vi "deflection reverse control.vi"() -> ()   [LabVIEW 2017]
uses:
  <vilib>/rvi/Emulation/niFpgaGetClockAttributes.vi
  <vilib>/rvi/Emulation/niFpgaSctlEmulationGetInTimedLoop.vi
  <vilib>/rvi/Emulation/niFpgaEmulationReportErrorSimple.vi
  <vilib>/rvi/eio/common/nirviEmuTemplateMethod_errors.vi
  <vilib>/rvi/Emulation/niFpgaCriticalErrorInLSC.vi
  <vilib>/eio/EIONode/EIONode.xnode
  <vilib>/rvi/FXPMathLib/FxpSub/XNode/nifxpmath_Sub.xnode
  <vilib>/rvi/FXPMathLib/FxpMul/XNode/nifxpmath_Multiplier.xnode
  <vilib>/rvi/FXPMathLib/FxpAdd/XNode/nifxpmath_Add.xnode
  <vilib>/rvi/FXPMathLib/sim/FxpSim.dll
panel:
  out "z sensor":fxp<+/-,20,5>
  in  "Lower Limit":fxp<+/-,64,29>=-8.0
  in  "Upper Limit":fxp<+/-,64,29>=8.0
  in  "P":fxp<+/-,20,5>=0.04998779296875
  in  "I":fxp<+/-,20,5>=0.029998779296875
  in  "SetPoint":fxp<+/-,20,5>
  in  "stop":bool
  out "deflection sensor":fxp<+/-,20,5>=0.018218994140625
  out "Output":fxp<+/-,64,29>=-1.1850092191016302
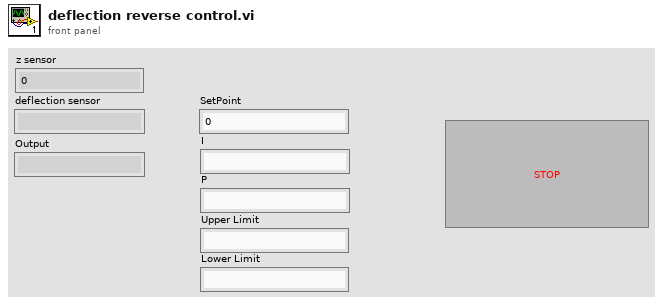
[diagram p1: front panel]
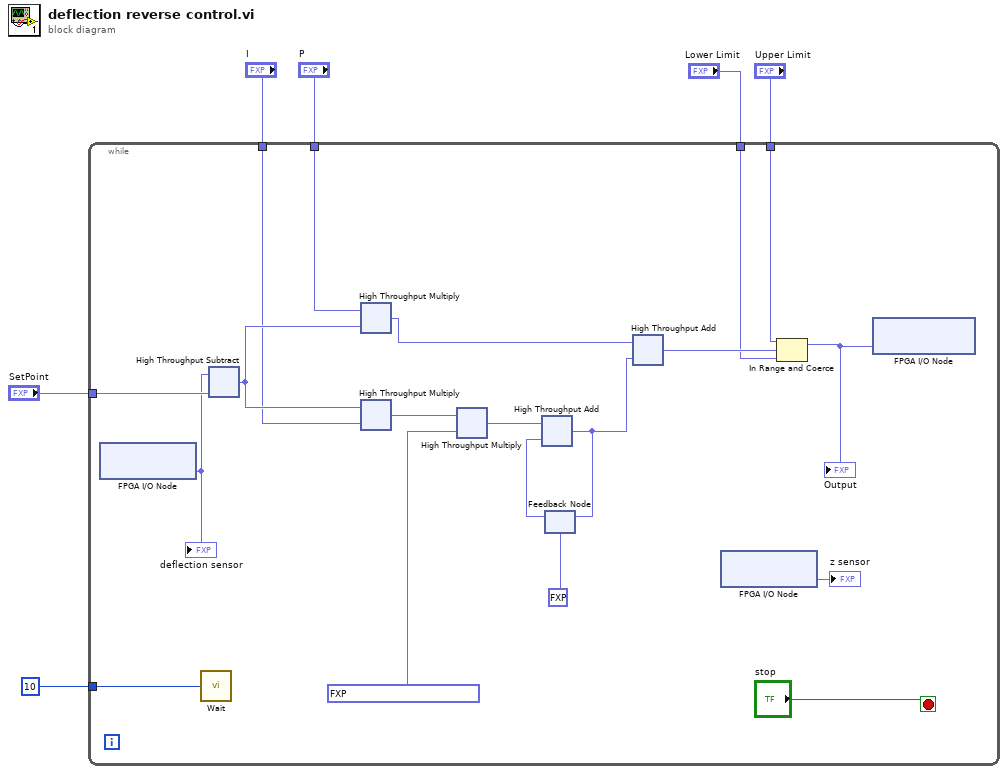
[diagram p0: block diagram]
diagram:
  n1 = while {
    tunnel: "SetPoint" -> [w9]
    tunnel: "P" -> [w24]
    tunnel: "I" -> [w22]
    tunnel: u32 10 ("Count(uSec)") -> [w20]
    tunnel: "Upper Limit" -> [w12]
    tunnel: "Lower Limit" -> [w11]
    stop <- "stop" stop-if-true
    n2 = xnode "FPGA I/O Node"() -> ("Mod1/AI3"=w8:fxp<+/-,20,5>)  [unwired: 1 in, 1 out]
    "deflection sensor" <- w8
    n3 = call "Wait"("Count(uSec)"=w20) -> ()  [unwired: 1 out]
    n4 = xnode ("High Throughput Subtract")("x"=w8, "y"=w9) -> ("x-y"=w23:fxp<+/-,21,6>)
    n5 = xnode ("High Throughput Multiply")("x"=w24, "y"=w23) -> ("x*y"=w15:fxp<+/-,41,11>)
    n6 = xnode ("High Throughput Multiply")("x"=w23, "y"=w22) -> ("x*y"=w21:fxp<+/-,41,11>)
    n7 = xnode ("High Throughput Multiply")("x"=w21, "y"=fxp<+/-,32,5> 9.998679161071777e-06) -> ("x*y"=w18:fxp<+/-,64,16>)
    n8 = feedback #1(fxp<+,1,1> 0.0) -> (w16:fxp<+/-,64,28>)
    n9 = xnode ("High Throughput Add")("x"=w18, "y"=w16) -> ("x+y"=w14:fxp<+/-,64,28>)
    n10 = feedback-in #1(w14) -> ()
    n11 = xnode ("High Throughput Add")("x"=w15, "y"=w14) -> ("x+y"=w13:fxp<+/-,64,29>)
    n12 = xnode "FPGA I/O Node"() -> ("Mod1/AI2"=→"z sensor":fxp<+/-,20,5>)  [unwired: 1 in, 1 out]
    n13 = In Range and Coerce(upper limit=w12, x=w13, lower limit=w11) -> (coerced(x)=w10:fxp<+/-,64,29>)  [unwired: 1 out]
    "Output" <- w10
    n14 = xnode "FPGA I/O Node"("Mod8/AO2"=w10) -> ()  [unwired: 1 in, 1 out]
  }
